vi "PC.vi"(11 "DataIn":T1) -> (3 "DataOut":T1)   [LabVIEW 2017]
doc: "SubVI criada para realizar a jogada do PC em caso de partida Player x PC"
uses:
  controls/DataIn.ctl
  controls/Tabuleiro.ctl
  controls/GameOption.ctl
  controls/Table.ctl
  controls/TabuleiroCoordenadas.ctl
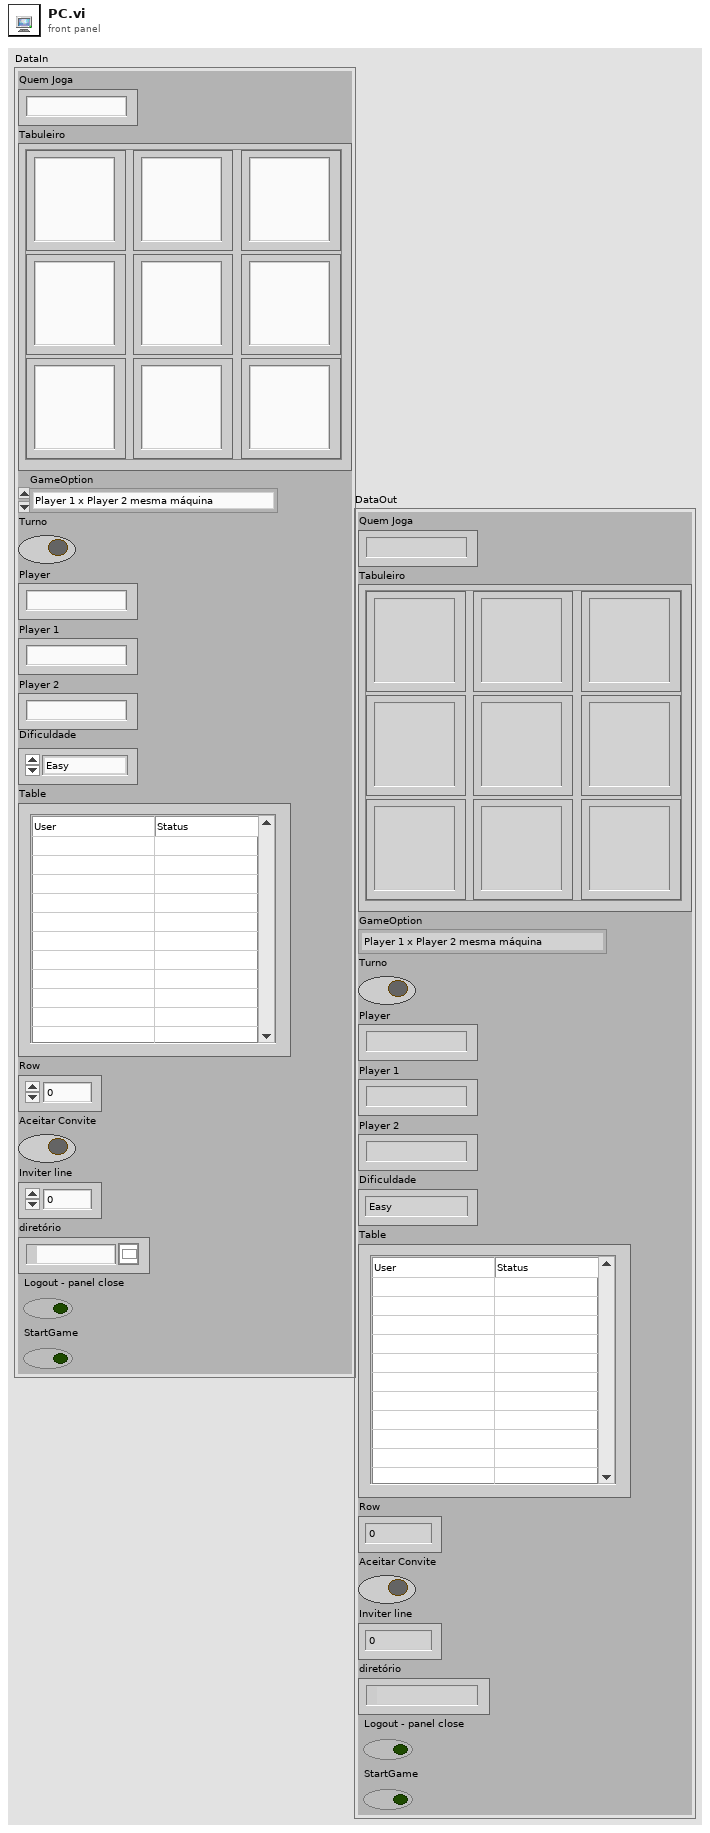
[diagram p1: front panel]
types:
  T1 = typedef "DataIn.ctl" = cluster{"Quem Joga":string, "Tabuleiro":T2, "GameOption":T3, "Turno":bool, "Player":string, "Player 1":string, "Player 2":string, "Dificuldade":enum16{"Easy", "Medium", "Hard"}, "Table":T4, "Row":u32, "Aceitar Convite":bool, "Inviter line":u32, "diretório":path, "Logout - panel close":bool, "StartGame":bool}
  T2 = typedef "Tabuleiro.ctl" = cluster{"(0,0)":string, "(1,0)":string, "(0,1)":string, "(1,1)":string, "(2,0)":string, "(1,2)":string, "(2,2)":string, "(0,2)":string, "(2,1) ":string}
  T3 = typedef "GameOption.ctl" = enum16{"Player 1 x Player 2 mesma máquina", "Player 1 x Player 2 pela rede", "Player 1 x Computador", "Wait for Event", "Initialize", "Stop"}
  T4 = typedef "Table.ctl" = string[][]
  T5 = typedef "TabuleiroCoordenadas.ctl" = enum16{"0,0", "0,1", "0,2", "1,0", "1,1", "1,2", "2,0", "2,1", "2,2"}
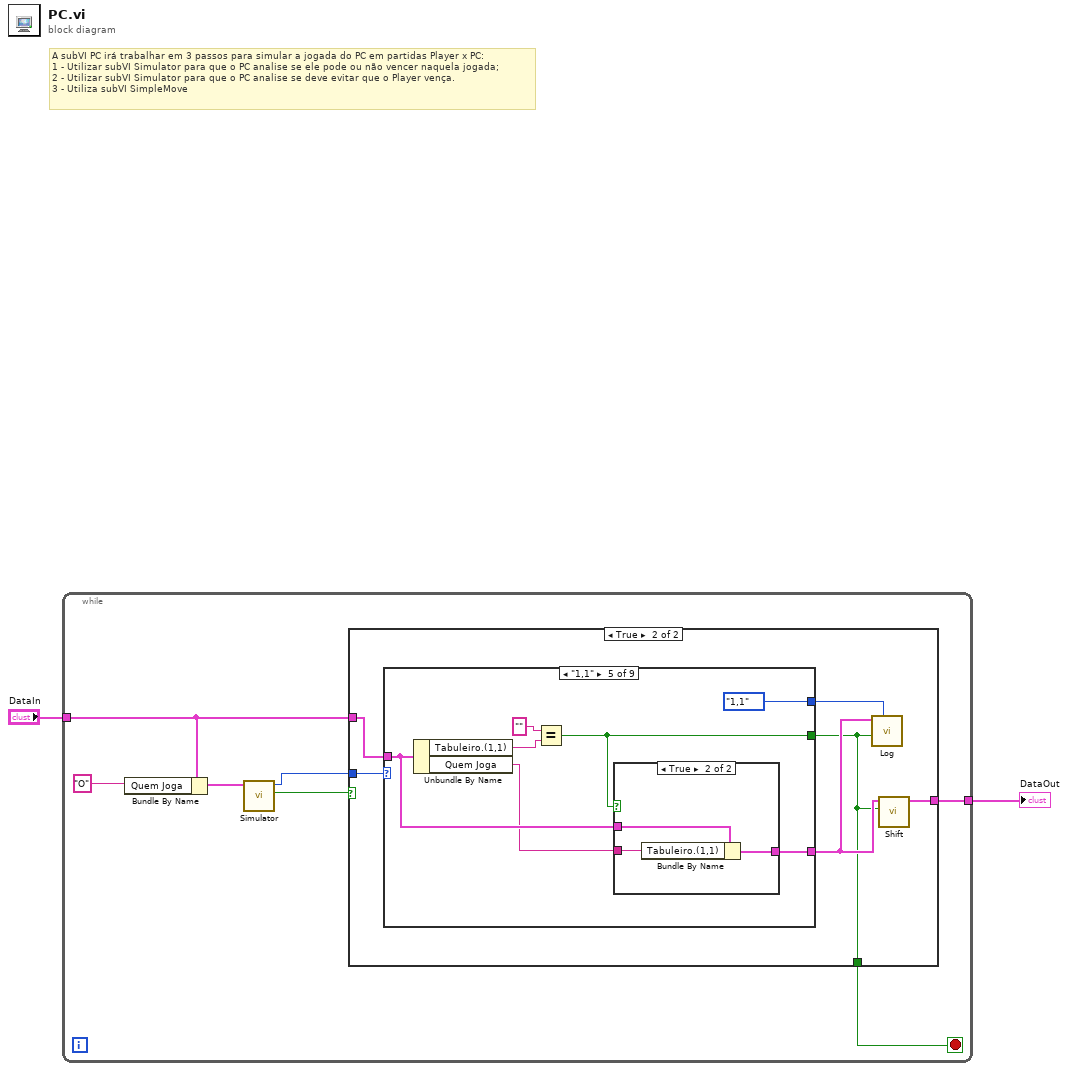
[diagram p0: block diagram]
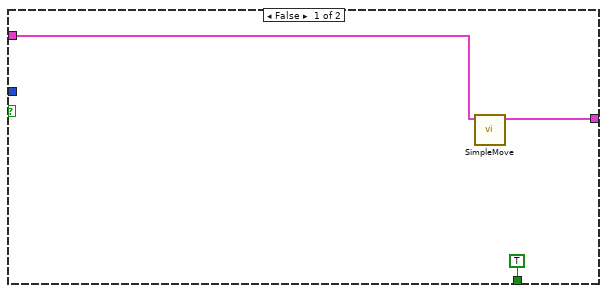
[diagram p2: hidden frame]
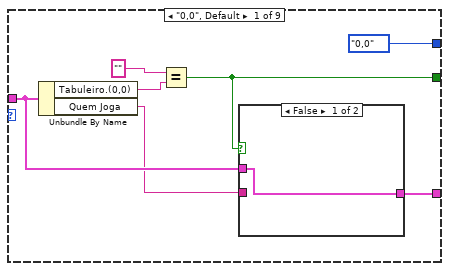
[diagram p3: hidden frame]
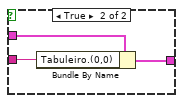
[diagram p4: hidden frame]
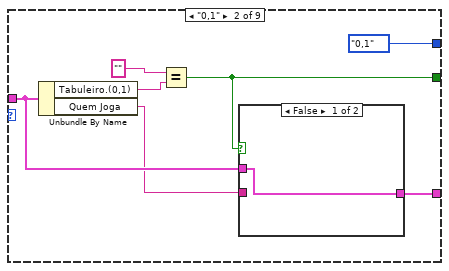
[diagram p5: hidden frame]
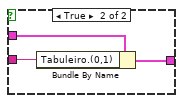
[diagram p6: hidden frame]
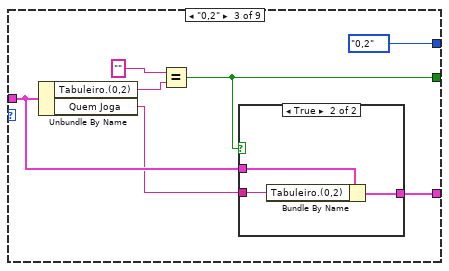
[diagram p7: hidden frame]
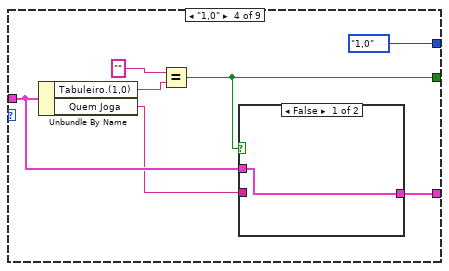
[diagram p9: hidden frame]
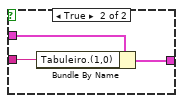
[diagram p10: hidden frame]
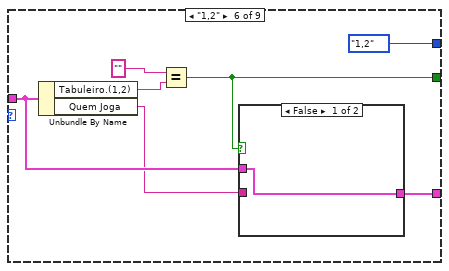
[diagram p12: hidden frame]
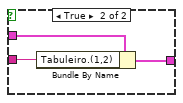
[diagram p13: hidden frame]
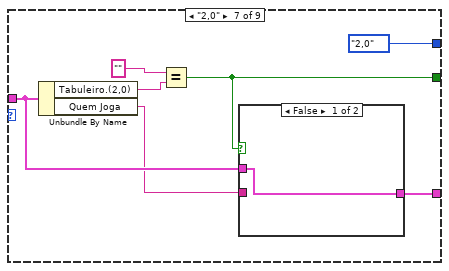
[diagram p14: hidden frame]
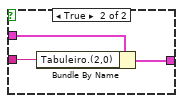
[diagram p15: hidden frame]
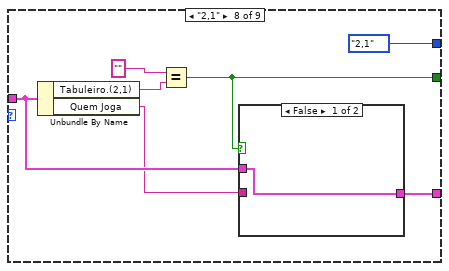
[diagram p16: hidden frame]
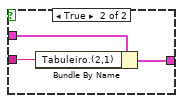
[diagram p17: hidden frame]
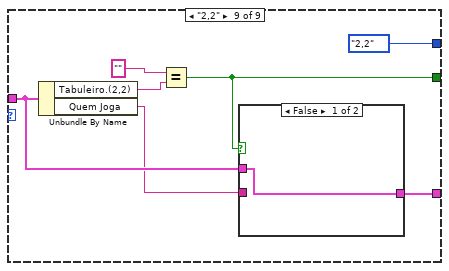
[diagram p18: hidden frame]
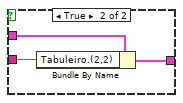
[diagram p19: hidden frame]
diagram:
  # "A subVI PC irá trabalhar em 3 passos para simular a jogada do PC em partidas Player x PC:\n1 - Utilizar subVI Simulator para que o PC analise se ele pode ou não vencer naquela jogada;\n2 - Utilizar subVI Simulator para que o PC analise se deve evitar que o Player vença.\n3 - Utiliza subVI SimpleMove"
  n1 = while {
    tunnel: "DataIn" -> [w9]
    tunnel: [w4] -> w1
    stop <- w3 stop-if-true
    n2 = Bundle By Name(cluster=w9, "Quem Joga"="O") -> (w6:T1)
    n3 = call "Simulator.vi"("DataIn"=w6) -> ("true = ganhou"=w7:bool, "Enum"=w8:T5)  [unwired: 9 in]
    n4 = case shown="True" w7 {
      tunnel: w8 -> [_ w18]
      tunnel: w9 -> [w11 w17]
      tunnel: [w12 w14] -> w4
      tunnel: [TRUE w13] -> w3
      frame False {
        n5 = call "SimpleMove.vi"("DataIn"=w11) -> ("DataOut"=w12:T1)  [unwired: 10 in]
      }
      frame True {
        n6 = case shown="\"1,1\"" w18 {
          tunnel: w17 -> [w22 w33 w44 w55 w66 w77 w88 w99 w110]
          tunnel: [w23 w34 w45 w56 w67 w78 w89 w100 w111] -> w13
          tunnel: [w20 w31 w42 w53 w64 w75 w86 w97 w108] -> w15
          tunnel: [TabuleiroCoordenadas."0,0" ("Enum") TabuleiroCoordenadas."0,1" ("Enum") TabuleiroCoordenadas."0,2" ("Enum") TabuleiroCoordenadas."1,0" ("Enum") TabuleiroCoordenadas."1,1" ("Enum") TabuleiroCoordenadas."1,2" ("Enum") TabuleiroCoordenadas."2,0" ("Enum") TabuleiroCoordenadas."2,1" ("Enum") TabuleiroCoordenadas."2,2" ("Enum")] -> w16
          frame "0,0", Default {
            n7 = Unbundle By Name(w22) -> ("Tabuleiro.(0,0)"=w25:string, "Quem Joga"=w21:string)
            n8 = Equal?(x="", y=w25) -> (x = y?=w23:bool)
            n9 = case shown="False" w23 {
              tunnel: w22 -> [w26 w29]
              tunnel: w21 -> [_ w28]
              tunnel: [w26 w27] -> w20
              frame False {
              }
              frame True {
                n10 = Bundle By Name(cluster=w29, "Tabuleiro.(0,0)"=w28) -> (w27:T1)
              }
            }
          }
          frame "0,1" {
            n11 = Unbundle By Name(w33) -> ("Tabuleiro.(0,1)"=w36:string, "Quem Joga"=w32:string)
            n12 = Equal?(x="", y=w36) -> (x = y?=w34:bool)
            n13 = case shown="False" w34 {
              tunnel: w33 -> [w37 w40]
              tunnel: w32 -> [_ w39]
              tunnel: [w37 w38] -> w31
              frame False {
              }
              frame True {
                n14 = Bundle By Name(cluster=w40, "Tabuleiro.(0,1)"=w39) -> (w38:T1)
              }
            }
          }
          frame "0,2" {
            n15 = Unbundle By Name(w44) -> ("Tabuleiro.(0,2)"=w47:string, "Quem Joga"=w43:string)
            n16 = Equal?(x="", y=w47) -> (x = y?=w45:bool)
            n17 = case shown="True" w45 {
              tunnel: w44 -> [w48 w51]
              tunnel: w43 -> [_ w50]
              tunnel: [w48 w49] -> w42
              frame False {
              }
              frame True {
                n18 = Bundle By Name(cluster=w51, "Tabuleiro.(0,2)"=w50) -> (w49:T1)
              }
            }
          }
          frame "1,0" {
            n19 = Unbundle By Name(w55) -> ("Tabuleiro.(1,0)"=w58:string, "Quem Joga"=w54:string)
            n20 = Equal?(x="", y=w58) -> (x = y?=w56:bool)
            n21 = case shown="False" w56 {
              tunnel: w55 -> [w59 w62]
              tunnel: w54 -> [_ w61]
              tunnel: [w59 w60] -> w53
              frame False {
              }
              frame True {
                n22 = Bundle By Name(cluster=w62, "Tabuleiro.(1,0)"=w61) -> (w60:T1)
              }
            }
          }
          frame "1,1" {
            n23 = Unbundle By Name(w66) -> ("Tabuleiro.(1,1)"=w69:string, "Quem Joga"=w65:string)
            n24 = Equal?(x="", y=w69) -> (x = y?=w67:bool)
            n25 = case shown="True" w67 {
              tunnel: w66 -> [w70 w73]
              tunnel: w65 -> [_ w72]
              tunnel: [w70 w71] -> w64
              frame False {
              }
              frame True {
                n26 = Bundle By Name(cluster=w73, "Tabuleiro.(1,1)"=w72) -> (w71:T1)
              }
            }
          }
          frame "1,2" {
            n27 = Unbundle By Name(w77) -> ("Tabuleiro.(1,2)"=w80:string, "Quem Joga"=w76:string)
            n28 = Equal?(x="", y=w80) -> (x = y?=w78:bool)
            n29 = case shown="False" w78 {
              tunnel: w77 -> [w81 w84]
              tunnel: w76 -> [_ w83]
              tunnel: [w81 w82] -> w75
              frame False {
              }
              frame True {
                n30 = Bundle By Name(cluster=w84, "Tabuleiro.(1,2)"=w83) -> (w82:T1)
              }
            }
          }
          frame "2,0" {
            n31 = Unbundle By Name(w88) -> ("Tabuleiro.(2,0)"=w91:string, "Quem Joga"=w87:string)
            n32 = Equal?(x="", y=w91) -> (x = y?=w89:bool)
            n33 = case shown="False" w89 {
              tunnel: w88 -> [w92 w95]
              tunnel: w87 -> [_ w94]
              tunnel: [w92 w93] -> w86
              frame False {
              }
              frame True {
                n34 = Bundle By Name(cluster=w95, "Tabuleiro.(2,0)"=w94) -> (w93:T1)
              }
            }
          }
          frame "2,1" {
            n35 = Unbundle By Name(w99) -> ("Tabuleiro.(2,1)"=w102:string, "Quem Joga"=w98:string)
            n36 = Equal?(x="", y=w102) -> (x = y?=w100:bool)
            n37 = case shown="False" w100 {
              tunnel: w99 -> [w103 w106]
              tunnel: w98 -> [_ w105]
              tunnel: [w103 w104] -> w97
              frame False {
              }
              frame True {
                n38 = Bundle By Name(cluster=w106, "Tabuleiro.(2,1)"=w105) -> (w104:T1)
              }
            }
          }
          frame "2,2" {
            n39 = Unbundle By Name(w110) -> ("Tabuleiro.(2,2)"=w113:string, "Quem Joga"=w109:string)
            n40 = Equal?(x="", y=w113) -> (x = y?=w111:bool)
            n41 = case shown="False" w111 {
              tunnel: w110 -> [w114 w117]
              tunnel: w109 -> [_ w116]
              tunnel: [w114 w115] -> w108
              frame False {
              }
              frame True {
                n42 = Bundle By Name(cluster=w117, "Tabuleiro.(2,2)"=w116) -> (w115:T1)
              }
            }
          }
        }
        n43 = call "Log.vi"("Enum Coordenadas"=w16, "Confirmação"=w13, "DataIn"=w15) -> ()  [unwired: 7 in, 2 out]
        n44 = call "Shift.vi"("Confirmação"=w13, "DataIn"=w15) -> ("DataOut"=w14:T1)  [unwired: 7 in, 2 out]
      }
    }
  }
  "DataOut" <- w1
